vi "创建参数二维码.vi"(11 "站点":string="站点测试") -> ()   [LabVIEW 2016, in "wxpusher.lvlib"]
uses:
  wxpusher.lvlib
  System.Windows.Forms
  <vilib>/Utility/miscctls.llb/LVPointTypeDef.ctl
  <vilib>/httpClient/POSTBuffer.vi
  <vilib>/httpClient/LabVIEWHTTPClient.lvlib
panel:
  out "url":string
  out "data.uid":string
  in  "测试":bool
  out "关注时间":string
  in  "关注信息":refnum<k24>(container) caption="黎山萧"
  in  "关闭":bool
  in  "带参数二维码":refnum<k24>(container)
  out "error out":errorcluster caption="错误输出"
  in  "error in (no error)":errorcluster caption="错误输入（无错误）"
  # "请使用微信扫描以下二维码"
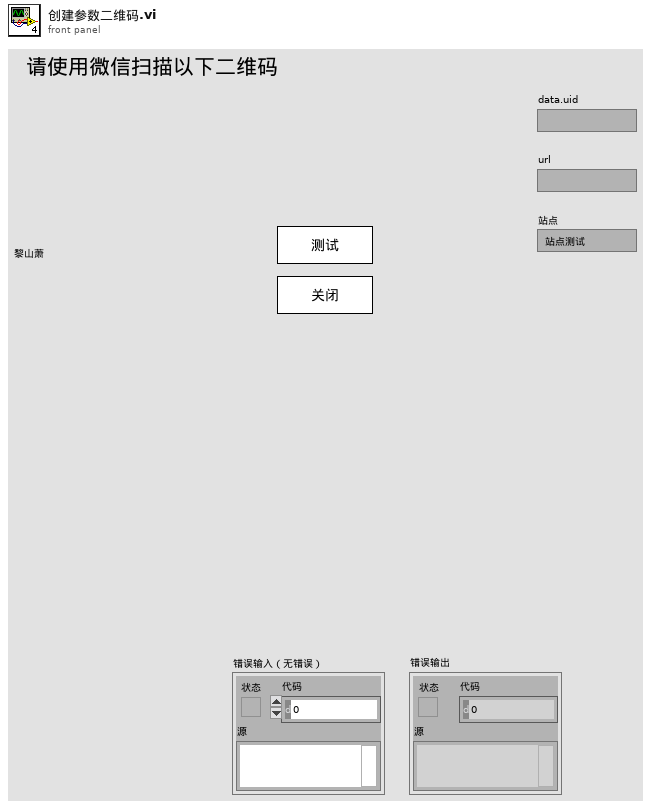
[diagram p1: front panel]
types:
  T1 = enum16{"初始化", "创建带参数二维码", "与服务器创建连接", "定时发送特征码", "接收回调信息", "处理回调信息", "展示关注信息", "结束"}[]
  T2 = enum16{"初始化", "创建带参数二维码", "与服务器创建连接", "定时发送特征码", "接收回调信息", "处理回调信息", "展示关注信息", "结束"}
  T3 = typedef "LVPointTypeDef.ctl" = cluster{"Horizontal":i16, "Vertical":i16}
  T4 = cluster{"code":u64, "msg":string, "data":cluster{"expires":u64, "code":string, "shortUrl":string, "extra":string, "url":string}, "success":bool}
  T5 = cluster{"appToken":string, "extra":string, "validTime":i32}
  T6 = enum16{"Standard", "Buffered", "CRLF", "Immediate"}
  T7 = cluster{"data":cluster{"action":string, "data":cluster{"appKey":string, "appName":string, "source":string, "time":u64, "uid":string, "userHeadImg":string, "userName":string, "extra":string}}}
  T8 = cluster{"cmd":string, "data":cluster{"png":u8[]}}
  T9 = typedef "LabVIEWHTTPClient.lvlib/ClientHandle.ctl" = refnum<k1>
  T10 = cluster{"expires":u64, "code":string, "shortUrl":string, "extra":string, "url":string}
  T11 = cluster{"action":string, "data":cluster{"appKey":string, "appName":string, "source":string, "time":u64, "uid":string, "userHeadImg":string, "userName":string, "extra":string}}
  T12 = cluster{"action":string, "data":cluster{"appKey":string, "appName":string, "source":string, "time":u64, "uid":string, "userHeadImg":string, "userName":string, "extra":string}}[]
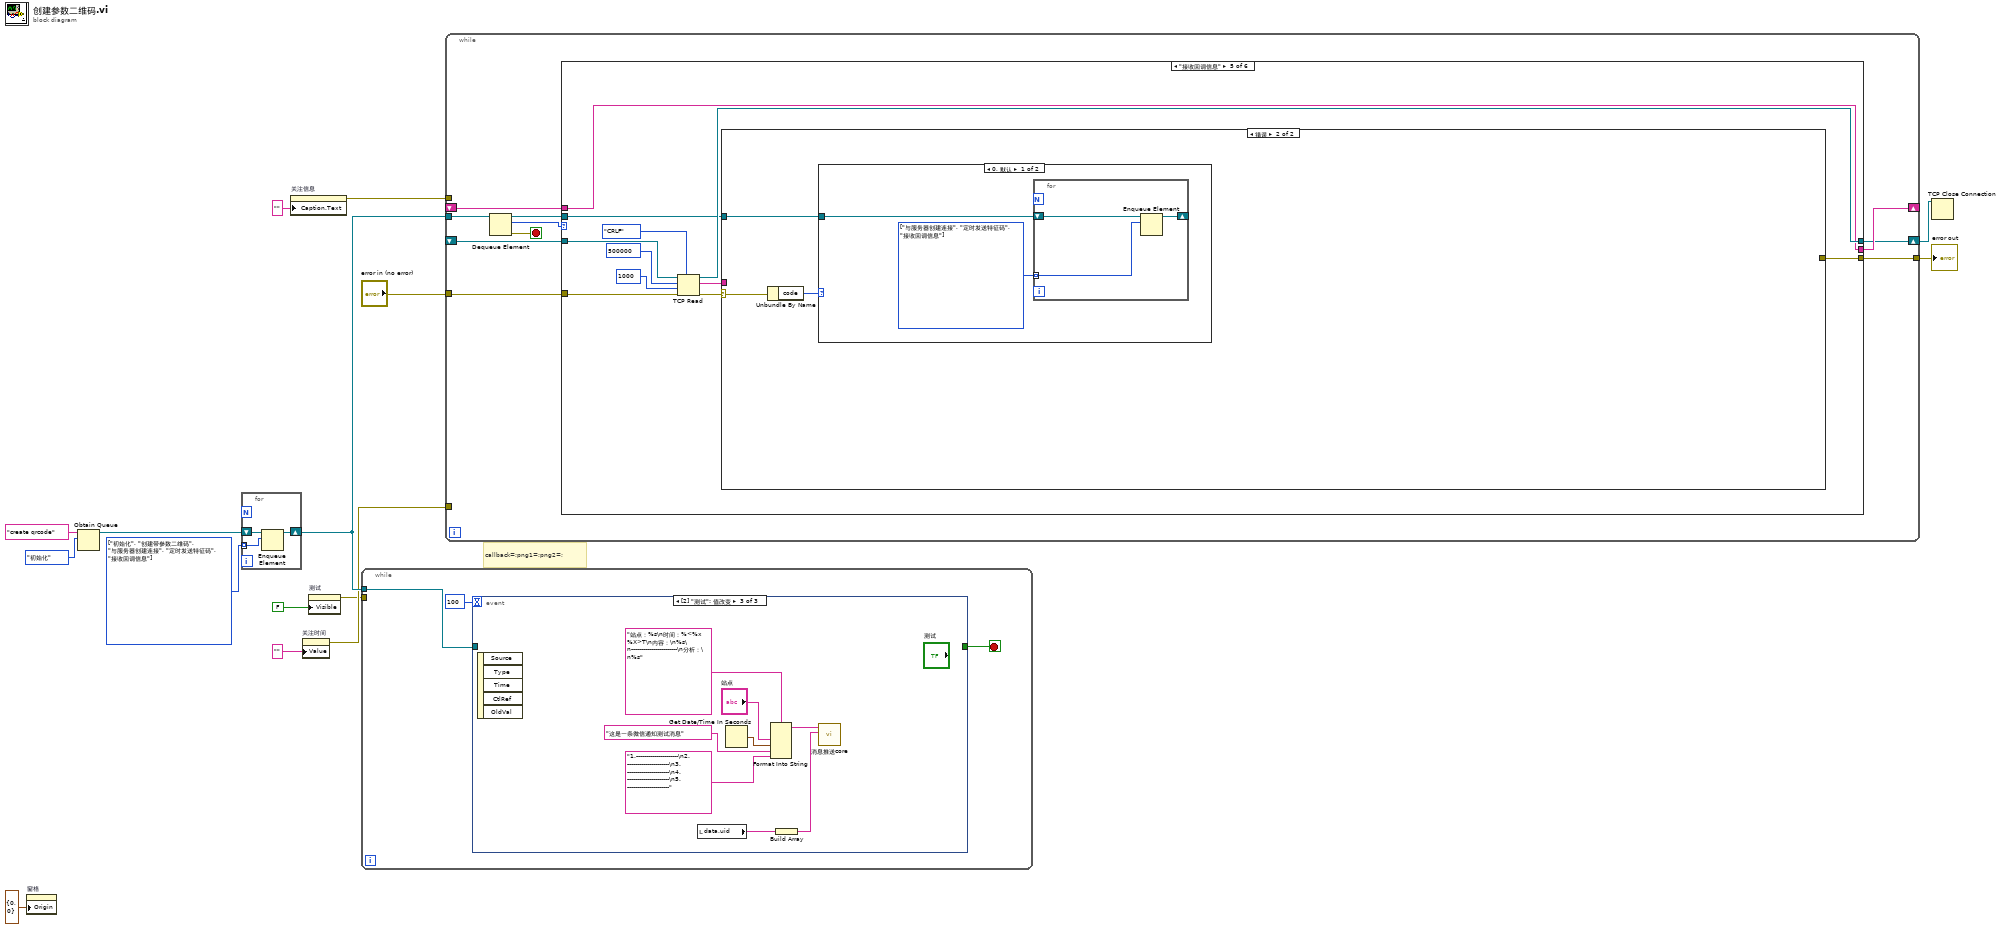
[diagram p0: block diagram]
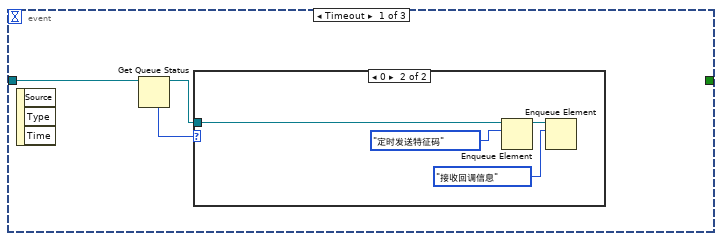
[diagram p2: hidden frame]
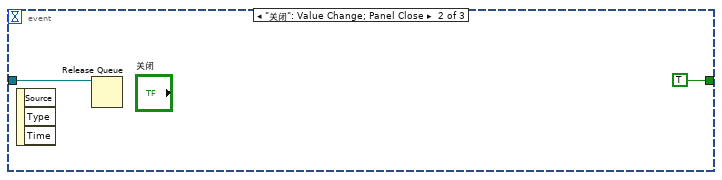
[diagram p4: hidden frame]
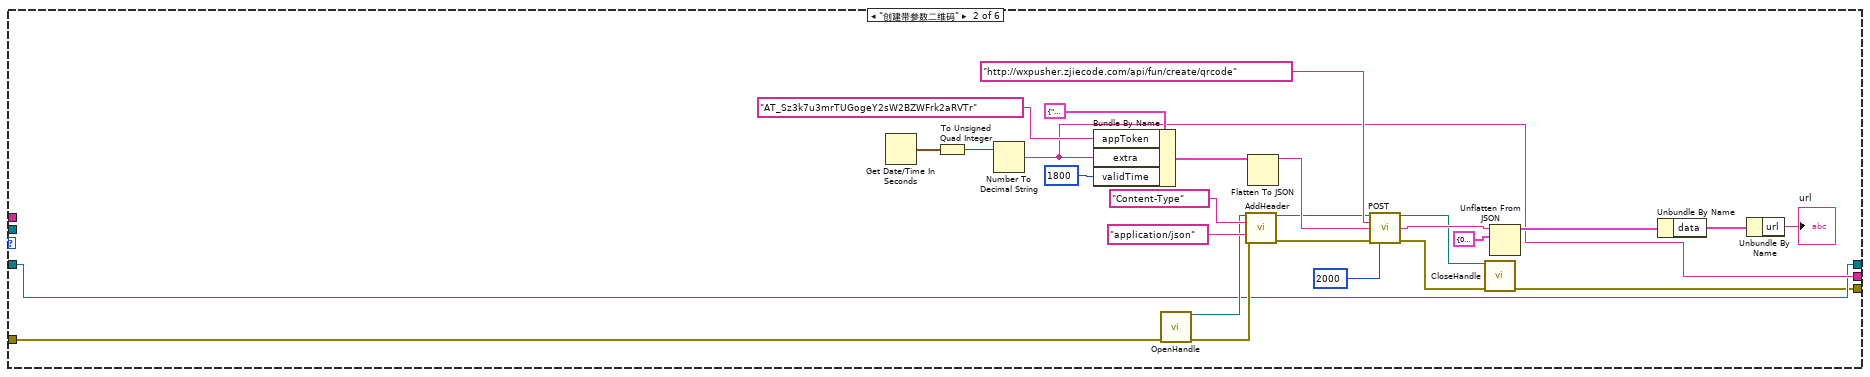
[diagram p6: hidden frame]
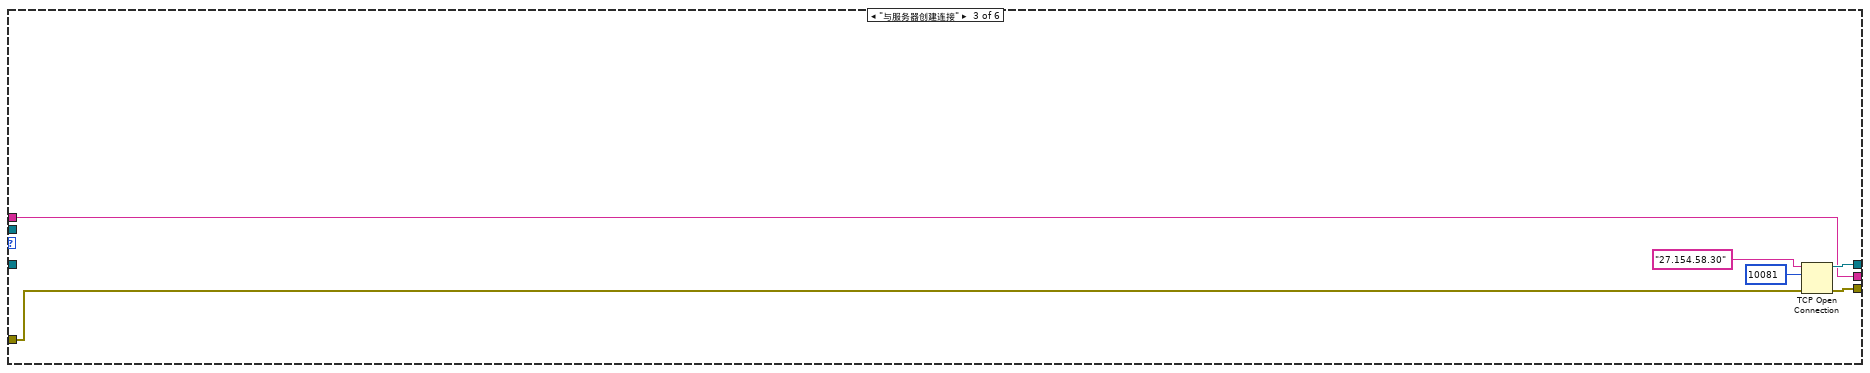
[diagram p7: hidden frame]
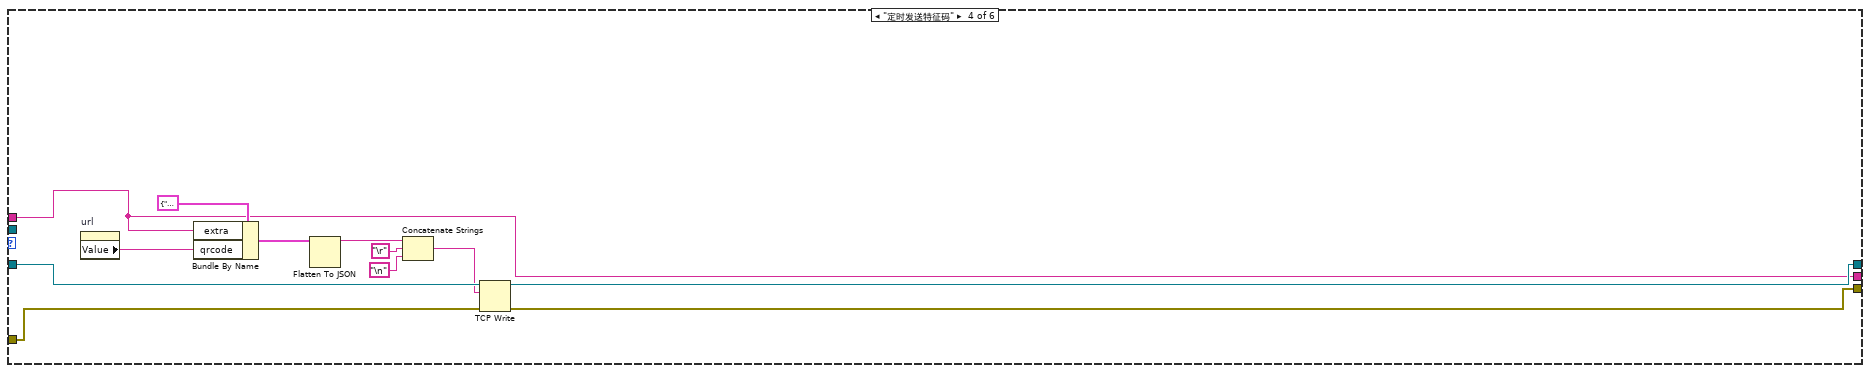
[diagram p8: hidden frame]
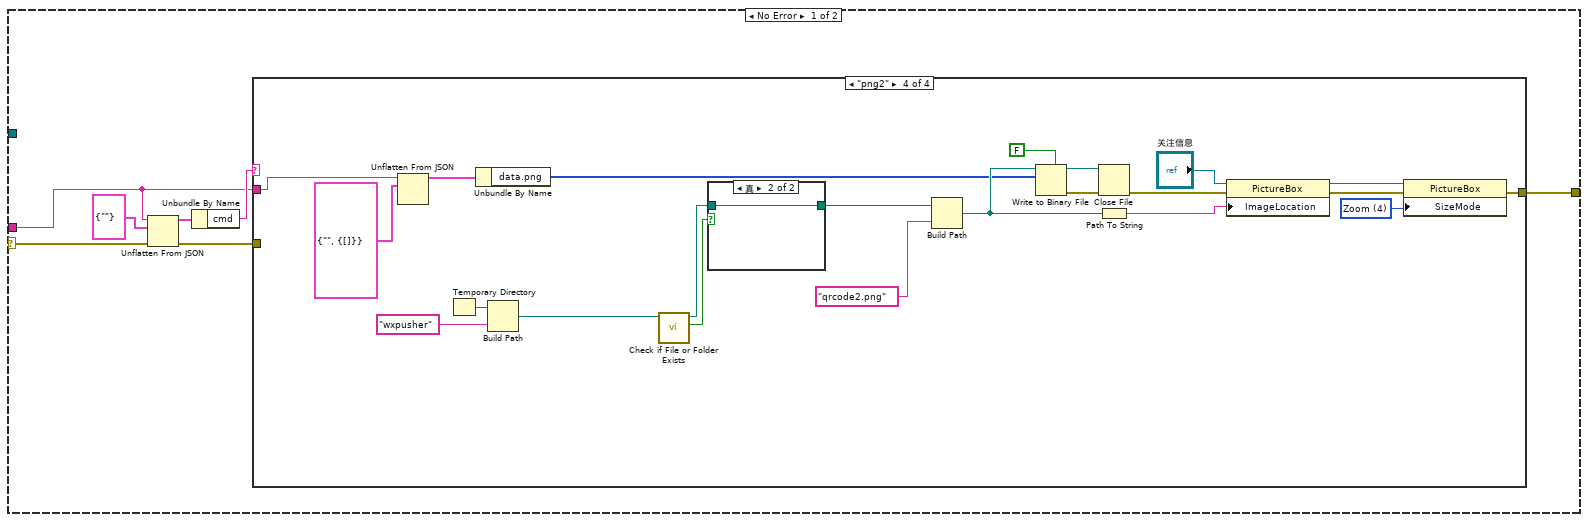
[diagram p9: hidden frame]
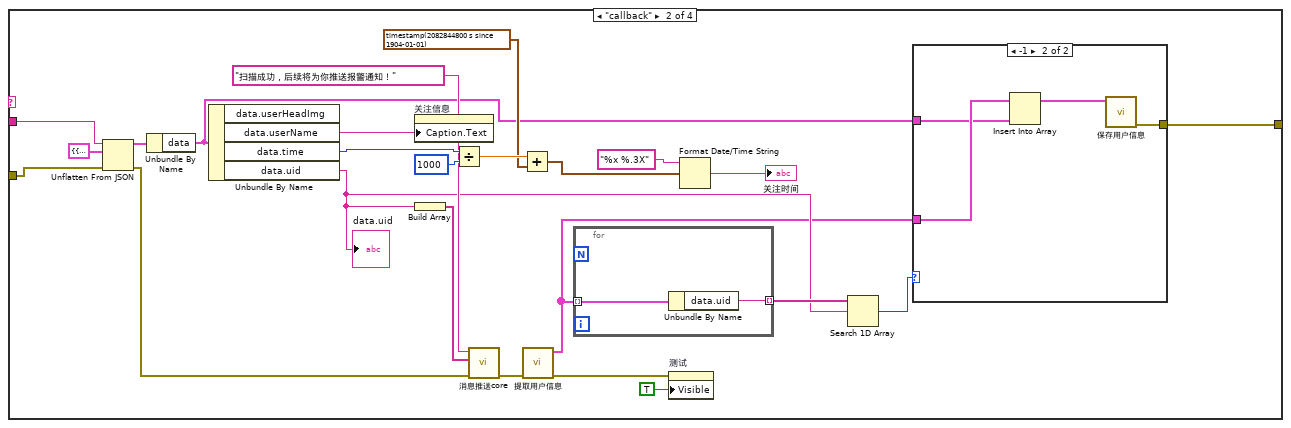
[diagram p11: hidden frame]
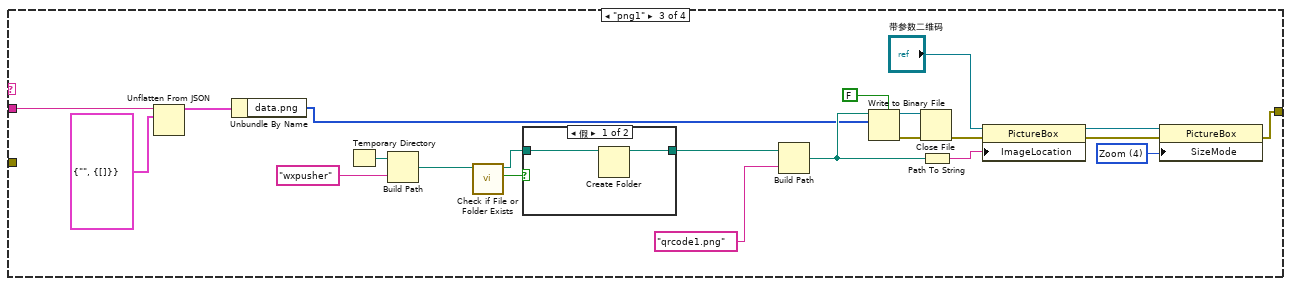
[diagram p13: hidden frame]
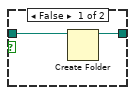
[diagram p15: hidden frame]
diagram:
  w8 = T1 [enum."初始化", enum."创建带参数二维码", enum."与服务器创建连接", enum."定时发送特征码", enum."接收回调信息"] items=["初始化", "创建带参数二维码", "与服务器创建连接", "定时发送特征码", "接收回调信息", "处理回调信息", "展示关注信息", "结束"]
  # "callback=;png1=;png2=;"
  n1 = property on="窗格" class="Pane"("Origin"=T3 {"Horizontal"=0, "Vertical"=0} ("原点")) -> ()  [unwired: 2 in, 2 out]
  n2 = Obtain Queue(name (unnamed)="create qrcode" ("名称（未命名）"), element data type=T2."初始化" ("枚举")) -> (queue out=w10:refnum<queue>)  [unwired: 3 in, 2 out]
  n3 = for {
    shift-right: [w17] -> w9
    shift-left: w10 -> [w18]
    tunnel: w8 -> [w16] mode=indexing
    n4 = Enqueue Element(queue=w18, element=w16) -> (queue out=w17:refnum<queue>)  [unwired: 2 in, 2 out]
  }
  n5 = property on="关注信息" class="AXCont"("Caption.Text"="" ("标题.文本")) -> (error out=w7:errorcluster)  [unwired: 2 in, 1 out]
  n6 = property on="关注时间" class="Str"("Value"="" ("关注时间")) -> (error out=w5:errorcluster)  [unwired: 2 in, 1 out]
  n7 = property on="测试" class="Bool"("Visible"=FALSE ("可见")) -> (error out=w1:errorcluster)  [unwired: 2 in, 1 out]
  n8 = while {
    tunnel: w9 -> [w20]
    tunnel: w1 -> [_]
    stop <- w21 stop-if-true
    n9 = event shown="[2] \"测试\": 值改变" {
      selector: _ -> [_ _ _]
      dyn-events: _ -> [_ _ _]
      timeout: 100 -> [_ _ _]
      tunnel: [_ TRUE _] -> w21
      tunnel: w20 -> [w24 w29 _]
      event Timeout {
        n10 = event-data() -> ()  [unwired: 1 in, 3 out]
        n11 = Get Queue Status(queue=w24) -> (queue out=w23:refnum<queue>, # elements in queue=w22:i32)  [unwired: 2 in, 6 out]
        n12 = case shown="0" w22 {
          tunnel: w23 -> [_ w25]
          frame Default {
          }
          frame 0 {
            n13 = Enqueue Element(queue=w25, element=T2."定时发送特征码" ("元素")) -> (queue out=w27:refnum<queue>)  [unwired: 2 in, 2 out]
            n14 = Enqueue Element(queue=w27, element=T2."接收回调信息" ("元素")) -> ()  [unwired: 2 in, 3 out]
          }
        }
      }
      event "关闭": Value Change; Panel Close {
        n15 = event-data() -> ()  [unwired: 1 in, 3 out]
        n16 = Release Queue(queue=w29) -> ()  [unwired: 2 in, 3 out]
      }
      event "测试": Value Change {
        n17 = event-data() -> ()  [unwired: 1 in, 5 out]
        n18 = local read "data.uid"() -> (w34:string)
        n19 = Get Date/Time In Seconds() -> (seconds since 1Jan1904=w32:timestamp)
        n20 = Format Into String(format string="站点：%s\n时间：%<%x %X>T\n内容：\n%s\n-----------------------\n分析：\n%s" ("格式字符串"), "站点", w32, "这是一条微信通知测试消息" ("内容"), "1.---------------------\n2.---------------------\n3.---------------------\n4.---------------------\n5.---------------------" ("分析")) -> (resulting string=w33:string)  [unwired: 2 in, 1 out]
        n21 = Build Array(w34) -> (w35:string[])
        n22 = call "消息推送core.vi"("数组"=w35, "content"=w33) -> ()  [unwired: 8 in, 2 out]
      }
    }
  }
  n23 = while {
    shift-right: [w48] -> _
    shift-left: _ -> [w47]
    tunnel: w9 -> [w46]
    tunnel: [w43] -> w12
    shift-right: [w44] -> w3
    shift-left: _ -> [w42]
    tunnel: "error in (no error)" -> [w41]
    tunnel: w7 -> [_]
    tunnel: w5 -> [_]
    stop <- w40 stop-if-true
    n24 = Dequeue Element(queue=w46) -> (queue out=w39:refnum<queue>, element=w45:T2, error out=w40:errorcluster)  [unwired: 2 in, 1 out]
    n25 = case shown="\"接收回调信息\"" w45 {
      tunnel: [w51 w59 w80 w90 w102 w203] -> w48
      tunnel: w47 -> [w51 _ w80 w90 w102 w203]
      tunnel: [w50 w58 w81 w95 w103 w202] -> w44
      tunnel: [w49 w52 w79 w94 w100 _] -> w43
      tunnel: w42 -> [w50 w58 _ w93 w104 w202]
      tunnel: w41 -> [w49 w57 w78 w92 w101 _]
      tunnel: w39 -> [_ _ _ _ w96 _]
      frame "初始化", Default {
      }
      frame "创建带参数二维码" {
        n26 = Get Date/Time In Seconds() -> (seconds since 1Jan1904=w74:timestamp)
        n27 = To Unsigned Quad Integer(1:w74) -> (0:w75:u64)
        n28 = Number To Decimal String(number=w75) -> (decimal integer string=w59:string)  [unwired: 1 in]
        n29 = Bundle By Name(cluster=T5 {"appToken"="", "extra"="", "validTime"=0}, "appToken"="AT_Sz3k7u3mrTUGogeY2sW2BZWFrk2aRVTr", "extra"=w59, "validTime"=1800 ("contentType")) -> (w70:T5)
        n30 = call <vilib>:"OpenHandle.vi"("error in (no error)"=w57) -> ("client handle out"=w60:T9, "error out"=w62:errorcluster)  [unwired: 13 in]
        n31 = call <vilib>:"AddHeader.vi"("client handle"=w60, "header"="Content-Type", "value"="application/json", "error in (no error)"=w62) -> ("client handle out"=w61:T9, "error out"=w65:errorcluster)  [unwired: 10 in]
        n32 = Flatten To JSON(anything=w70) -> (JSON string=w71:string)  [unwired: 2 in, 1 out]
        n33 = call-poly <vilib>:"POST.vi"("client handle"=w61, "url"="http://wxpusher.zjiecode.com/api/fun/create/qrcode", "buffer"=w71, "error in (no error)"=w65, "timeout (10000)"=2000) -> ("client handle out"=w53:T9, "body"=w72:string, "error out"=w54:errorcluster)  [unwired: 7 in, 1 out]
        n34 = call <vilib>:"CloseHandle.vi"("client handle"=w53, "error in (no error)"=w54) -> ("error out"=w52:errorcluster)  [unwired: 13 in]
        n35 = Unflatten From JSON(JSON string=w72, type and defaults=T4 {"code"=0, "msg"="", "data"={"expires"=0, "code"="", "shortUrl"="", "extra"="", "url"=""}, "success"=FALSE}) -> (value=w77:T4)  [unwired: 5 in, 1 out]
        n36 = Unbundle By Name(w77) -> ("data"=w76:T10)
        n37 = Unbundle By Name(w76) -> ("url"=→"url":string)
      }
      frame "与服务器创建连接" {
        n38 = TCP Open Connection(address="27.154.58.30" ("地址"), remote port or service name=u16 10081 ("远程端口或服务名称"), error in (no error)=w78) -> (connection ID=w81:refnum<k5>, error out=w79:errorcluster)  [unwired: 2 in]
      }
      frame "定时发送特征码" {
        n39 = property on="url" class="Str"() -> ("Value"=w89:string)  [unwired: 2 in, 2 out]
        n40 = Bundle By Name(cluster=cluster{"extra":string, "qrcode":string} {"extra"="", "qrcode"=""}, "extra"=w90, "qrcode"=w89) -> (w86:cluster{"extra":string, "qrcode":string})
        n41 = Flatten To JSON(anything=w86) -> (JSON string=w85:string)  [unwired: 2 in, 1 out]
        n42 = Concatenate Strings(w85, "\r", "\n") -> (w84:string)
        n43 = TCP Write(connection ID=w93, data in=w84, error in (no error)=w92) -> (connection ID out=w95:refnum<k5>, error out=w94:errorcluster)  [unwired: 1 in, 1 out]
      }
      frame "接收回调信息" {
        n44 = TCP Read(connection ID=w104, bytes to read=500000 ("读取的字节"), error in (no error)=w101, 7:T6."CRLF" ("模式（标准）"), 9:1000 ("超时毫秒(25000)")) -> (connection ID out=w103:refnum<k5>, data out=w106:string, error out=w98:errorcluster)
        n45 = case shown="错误" w98 {
          selector: w98 -> [w108 w196]
          tunnel: [w113 _] -> w100
          tunnel: w106 -> [w109 _]
          tunnel: w96 -> [_ w194]
          frame No Error {
            n46 = Unflatten From JSON(JSON string=w109, type and defaults=cluster{"cmd":string} {"cmd"=""}, error in (no error)=w108) -> (value=w111:cluster{"cmd":string}, error out=w107:errorcluster)  [unwired: 4 in]
            n47 = Unbundle By Name(w111) -> ("cmd"=w110:string)
            n48 = case shown="\"png2\"" w110 {
              tunnel: [_ w121 w149 w180] -> w113
              tunnel: w107 -> [_ w120 _ _]
              tunnel: w109 -> [_ w116 w147 w172]
              frame "假", Default {
              }
              frame "callback" {
                n49 = Unflatten From JSON(JSON string=w116, type and defaults=T7 {"data"={"action"="", "data"={"appKey"="", "appName"="", "source"="", "time"=0, "uid"="", "userHeadImg"="", "userName"="", "extra"=""}}} ("输出簇"), error in (no error)=w120) -> (value=w118:T7, error out=w129:errorcluster)  [unwired: 4 in]
                n50 = Unbundle By Name(w118) -> ("data"=w117:T11)
                n51 = Unbundle By Name(w117) -> ("data.userName"=w130:string, "data.time"=w137:u64, "data.uid"=w125:string)  [unwired: 1 out]
                "data.uid" <- w125
                n52 = property on="关注信息" class="AXCont"("Caption.Text"=w130) -> ()  [unwired: 2 in, 2 out]
                n53 = Build Array(w125) -> (w127:string[])
                n54 = Divide(x=w137, y=u64 1000) -> (x/y=w135:dbl)
                n55 = call "消息推送core.vi"("error in (no error)"=w129, "数组"=w127, "content"="扫描成功，后续将为你推送报警通知！") -> ("error out"=w122:errorcluster)  [unwired: 7 in, 1 out]
                n56 = Add(x=w135, y=timestamp(2082844800 s since 1904-01-01)) -> (x+y=w133:timestamp)
                n57 = call "提取用户信息.vi"("error in (no error)"=w122) -> ("error out"=w114:errorcluster, "用户信息"=w123:T12)  [unwired: 9 in]
                n58 = for {
                  tunnel: w123 -> [w143] mode=indexing
                  tunnel: [w142] -> w126 mode=indexing
                  n59 = Unbundle By Name(w143) -> ("data.uid"=w142:string)
                }
                n60 = property on="测试" class="Bool"(error in=w114, "Visible"=TRUE ("可见")) -> ()  [unwired: 1 in, 2 out]
                n61 = Format Date/Time String(time format string (%c)="%x %.3X" ("时间格式字符串(%c)"), seconds (now)=w133) -> (date/time string=→"关注时间":string)  [unwired: 1 in]
                n62 = Search 1D Array(1D array=w126, element=w125) -> (index of element=w124:i32)  [unwired: 1 in]
                n63 = case shown="-1" w124 {
                  tunnel: w123 -> [_ w141]
                  tunnel: w117 -> [_ w140]
                  tunnel: [_ w138] -> w121
                  frame 0, Default {
                  }
                  frame -1 {
                    n64 = Insert Into Array(array=w141, new element=w140) -> (w139:T12)  [unwired: 1 in]
                    n65 = call "保存用户信息.vi"("用户信息"=w139) -> ("error out"=w138:errorcluster)  [unwired: 10 in]
                  }
                }
              }
              frame "png1" {
                w156 = 4 items=["Normal", "StretchImage", "AutoSize", "CenterImage", "Zoom"] ("SizeMode")
                n66 = Unflatten From JSON(JSON string=w147, type and defaults=T8 {"cmd"="", "data"={"png"=[]}}) -> (value=w146:T8)  [unwired: 5 in, 1 out]
                n67 = Unbundle By Name(w146) -> ("data.png"=w145:u8[])
                n68 = Temporary Directory() -> (w165:path)
                n69 = Build Path(base path=w165, name or relative path="wxpusher" ("名称或相对路径")) -> (appended path=w160:path)
                n70 = call <vilib>:"Check if File or Folder Exists.vi"("path"=w160) -> ("file or folder exists?"=w163:bool, "dup path"=w162:path)  [unwired: 8 in, 1 out]
                n71 = case shown="假" w163 {
                  tunnel: [w166 w168] -> w159
                  tunnel: w162 -> [w167 w168]
                  frame False {
                    n72 = Create Folder(path (use dialog)=w167) -> (created path=w166:path)  [unwired: 2 in, 2 out]
                  }
                  frame True {
                  }
                }
                n73 = Build Path(base path=w159, name or relative path="qrcode1.png" ("名称或相对路径")) -> (appended path=w151:path)
                n74 = Write to Binary File(file (use dialog)=w151, data=w145, 5:FALSE ("预置数组或字符串大小？ (T)")) -> (refnum out=w158:refnum<file>, error out=w157:errorcluster)  [unwired: 3 in, 1 out]
                n75 = Close File(refnum=w158, error in=w157) -> (error out=w150:errorcluster)  [unwired: 1 out]
                n76 = Path To String(path=w151) -> (string=w152:string)
                n77 = property on="属性节点" class="PictureBox"(reference="带参数二维码", error in=w150, "ImageLocation"=w152) -> (reference out=w155:refnum<k24>, error out=w153:errorcluster)
                n78 = property class="PictureBox"(reference=w155, error in=w153, "SizeMode"=w156) -> (error out=w149:errorcluster)  [unwired: 1 out]
              }
              frame "png2" {
                w188 = 4 items=["Normal", "StretchImage", "AutoSize", "CenterImage", "Zoom"] ("SizeMode")
                n79 = Unflatten From JSON(JSON string=w172, type and defaults=T8 {"cmd"="", "data"={"png"=[]}}) -> (value=w173:T8)  [unwired: 5 in, 1 out]
                n80 = Temporary Directory() -> (w179:path)
                n81 = Unbundle By Name(w173) -> ("data.png"=w171:u8[])
                n82 = Build Path(base path=w179, name or relative path="wxpusher" ("名称或相对路径")) -> (appended path=w175:path)
                n83 = call <vilib>:"Check if File or Folder Exists.vi"("path"=w175) -> ("file or folder exists?"=w177:bool, "dup path"=w176:path)  [unwired: 8 in, 1 out]
                n84 = case shown="真" w177 {
                  tunnel: [w191 w193] -> w174
                  tunnel: w176 -> [w192 w193]
                  frame False {
                    n85 = Create Folder(path (use dialog)=w192) -> (created path=w191:path)  [unwired: 2 in, 2 out]
                  }
                  frame True {
                  }
                }
                n86 = Build Path(base path=w174, name or relative path="qrcode2.png" ("名称或相对路径")) -> (appended path=w182:path)
                n87 = Write to Binary File(file (use dialog)=w182, data=w171, 5:FALSE ("预置数组或字符串大小？ (T)")) -> (refnum out=w185:refnum<file>, error out=w186:errorcluster)  [unwired: 3 in, 1 out]
                n88 = Close File(refnum=w185, error in=w186) -> (error out=w184:errorcluster)  [unwired: 1 out]
                n89 = Path To String(path=w182) -> (string=w181:string)
                n90 = property on="属性节点" class="PictureBox"(reference="关注信息", error in=w184, "ImageLocation"=w181) -> (reference out=w189:refnum<k24>, error out=w183:errorcluster)
                n91 = property class="PictureBox"(reference=w189, error in=w183, "SizeMode"=w188) -> (error out=w180:errorcluster)  [unwired: 1 out]
              }
            }
          }
          frame Error {
            n92 = Unbundle By Name(w196) -> ("code"=w195:i32)
            n93 = case shown="0, 默认" w195 {
              tunnel: w194 -> [w197 _]
              frame 0, Default {
                w198 = T1 [enum."与服务器创建连接", enum."定时发送特征码", enum."接收回调信息"] items=["初始化", "创建带参数二维码", "与服务器创建连接", "定时发送特征码", "接收回调信息", "处理回调信息", "展示关注信息", "结束"]
                n94 = for {
                  shift-right: [w200] -> _
                  shift-left: w197 -> [w201]
                  tunnel: w198 -> [w199] mode=indexing
                  n95 = Enqueue Element(queue=w201, element=w199) -> (queue out=w200:refnum<queue>)  [unwired: 2 in, 2 out]
                }
              }
              frame 56 {
              }
            }
          }
        }
      }
      frame "结束" {
      }
    }
  }
  "error out" <- w12
  n96 = TCP Close Connection(connection ID=w3) -> ()  [unwired: 2 in, 2 out]
